vi "Ev i.vi"(8 "error in (no error)":errorcluster, 11 "IDE simple in":refnum<class "Main Panel.lvclass">) -> (0 "error out":errorcluster, 3 "IDE simple out":refnum<class "Main Panel.lvclass">)   [LabVIEW 2018, in "Main Panel.lvlib" / "Main Panel.lvclass"]
uses:
  Main Panel.lvclass
  Main Panel.lvclass/Main Panel.ctl
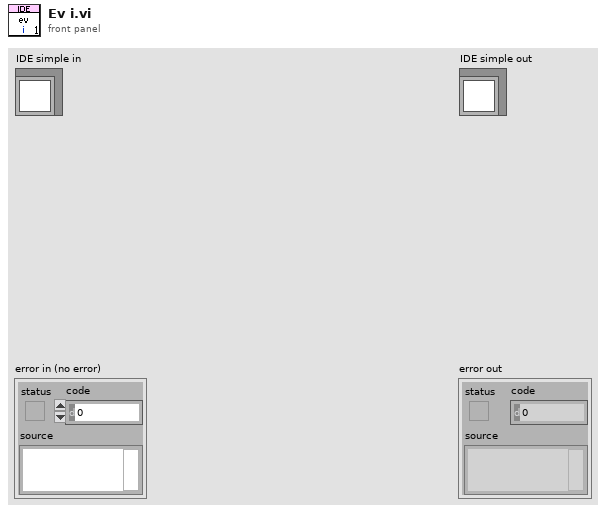
[diagram p1: front panel]
types:
  T1 = typedef "Data Parser.lvclass/frame i data.ctl" = cluster{"kind":string, "x":string, "y":string, "w":string, "h":string, "dvx":string, "dvy":string, "dvz":string, "fall":string, "arest":string, "vrest":string, "bdefend":string, "injury":string, "zwidth":string, "effect":string, "catchingact":string, "caughtact":string}
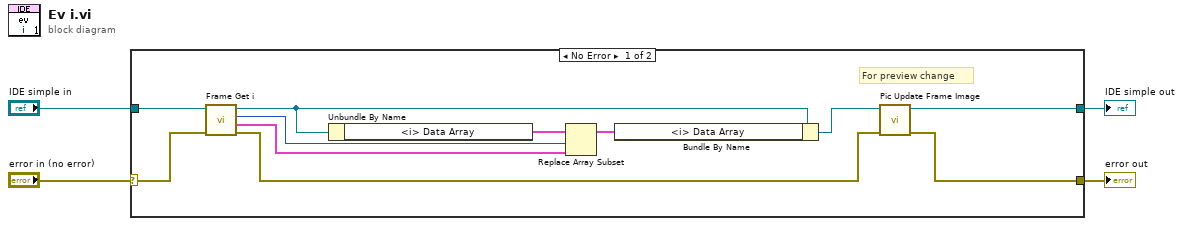
[diagram p0: block diagram]
diagram:
  n1 = case shown="No Error" "error in (no error)" {
    selector: "error in (no error)" -> [w14 w17]
    tunnel: [w5 w17] -> w3
    tunnel: [w6 w16] -> w1
    tunnel: "IDE simple in" -> [w15 w16]
    frame No Error {
      # "For preview change"
      n2 = call "Frame Get i.vi"("error in (no error)"=w14, "IDE simple in"=w15) -> ("error out"=w7:errorcluster, "<i> Data"=w9:T1, "Iindex"=w10:u32, "IDE simple out"=w13:refnum<class "Main Panel.lvclass">)  [unwired: 6 in]
      n3 = Unbundle By Name(w13) -> ("<i> Data Array"=w12:T1[])
      n4 = Replace Array Subset(array=w12, new element=w9, index=w10) -> (w11:T1[])
      n5 = Bundle By Name(cluster=w13, "<i> Data Array"=w11) -> (w8:refnum<class "Main Panel.lvclass">)
      n6 = call "Pic Update Frame Image.vi"("error in (no error)"=w7, "LF2R IDE in"=w8) -> ("error out"=w5:errorcluster, "LF2R IDE out"=w6:refnum<class "Main Panel.lvclass">)  [unwired: 8 in]
    }
    frame Error {
    }
  }
  "error out" <- w3
  "IDE simple out" <- w1
